vi "Untitled 4 (SubVI).vi"(11 "Numeric":dbl) -> (3 "PT100":dbl)   [LabVIEW 2017]
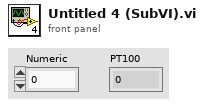
[diagram p1: front panel]
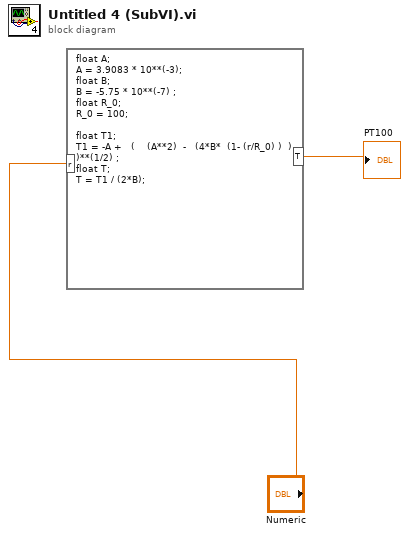
[diagram p0: block diagram]
diagram:
  n1 = formula code="float A;\nA = 3.9083 * 10**(-3);\nfloat B;\nB = -5.75 * 10**(-7) ;\nfloat R_0;\nR_0 = 100;\n\nfloat T1;\nT1 = -A +   (    (A**2)  -   (4*B*  (1- (r/R_0) )  )      )**(1/2) ;\nfloat T;  \nT = T1 / (2*B);"("r"="Numeric") -> ("T"=→"PT100":dbl)
